vi "Do.vi"(8 "error in (no error)":errorcluster, 10 "Actor in":refnum<class "Actor.lvclass">, 11 "Configure Output Mode Msg":refnum<class "Configure Output Mode Msg.lvclass">) -> (0 "error out":errorcluster, 2 "Actor out":refnum<class "Actor.lvclass">)   [LabVIEW 2015, in "CS++Fgen.lvlib" / "Configure Output Mode Msg.lvclass"]
doc: "This VI delivers the message to the actor by calling the appropriate method(s) on the actor."
uses:
  Configure Output Mode Msg.lvclass
  <vilib>/ActorFramework/Actor/Actor.lvclass
  CS++Fgen/CS++Fgen.lvclass
  CSPP_Core/Actors/CS++PVMonitor Messages/CS++PVUpdate Msg/CS++PVUpdate Msg.lvclass/CS++PVUpdate Msg.ctl
  CSPP_Core/Classes/CS++ProcessVariables/ProcessVariable/PV.lvclass/PV.ctl
  Configure Output Mode Msg.lvclass/Configure Output Mode Msg.ctl
  CSPP_Core/Classes/CS++ProcessVariables/ProcessVariable/PV.lvclass
  CSPP_Core/Actors/CS++PVMonitor Messages/CS++PVUpdate Msg/CS++PVUpdate Msg.lvclass
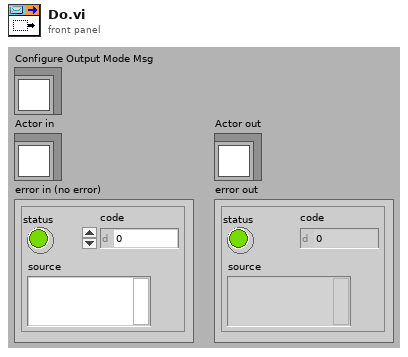
[diagram p1: front panel]
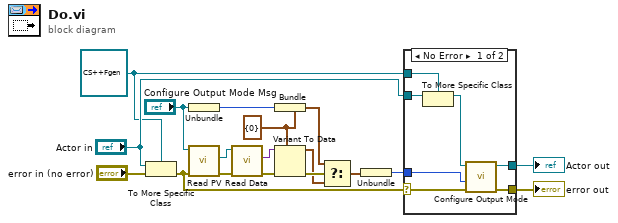
[diagram p0: block diagram]
diagram:
  w10 = cluster{"output mode (Standard Function)":i32} {"output mode (Standard Function)"=0} ("Type")
  w14 = refnum<class "CS++Fgen.lvclass"> refnum ("Actor in")
  n1 = To More Specific Class(target class=w14, reference="Actor in", error in="error in (no error)") -> (error out=w3:errorcluster)  [unwired: 1 out]
  n2 = Unbundle ("Pre-Unbundler")("Configure Output Mode Msg") -> (w1:i32)
  n3 = call "Read PV.vi"("error in (no error)"=w3, "CS++PVUpdate Msg in"="Configure Output Mode Msg") -> ("error out"=w13:errorcluster, "PV"=w9:refnum<class "PV.lvclass">)  [unwired: 7 in, 1 out]
  n4 = call "Read Data.vi"("error in (no error)"=w13, "PV in"=w9) -> ("error out"=w7:errorcluster, "Data"=w8:variant)  [unwired: 7 in, 1 out]
  n5 = Bundle ("Pre-Bundler")(cluster=w10, "output mode (Standard Function)"=w1) -> (w11:cluster{"output mode (Standard Function)":i32})
  n6 = Variant To Data(error in=w7, type=w10, Variant=w8) -> (data=w5:cluster{"output mode (Standard Function)":i32}, error out=w12:errorcluster)
  n7 = Select ("MainSelect")(t=w11, s=w12, f=w5) -> (s? t:f=w6:cluster{"output mode (Standard Function)":i32})
  n8 = Unbundle ("Main-Unbundler")(w6) -> ("output mode (Standard Function)"=w2:i32)
  n9 = case shown="No Error" w3 {
    selector: w3 -> [w23 w27]
    tunnel: [w25 w27] -> w17
    tunnel: [w24 w26] -> w16
    tunnel: "Actor in" -> [w22 w26]
    tunnel: w14 -> [w21 _]
    tunnel: w2 -> [w19 _]
    frame No Error {
      n10 = To More Specific Class(target class=w21, reference=w22) -> (specific class reference=w20:refnum<class "CS++Fgen.lvclass">)  [unwired: 1 in, 1 out]
      n11 = call "Configure Output Mode.vi"("error in (no error)"=w23, "output mode (Standard Function)"=w19, "CS++Fgen in"=w20) -> ("error out"=w25:errorcluster, "CS++Fgen out"=w24:refnum<class "CS++Fgen.lvclass">)  [unwired: 7 in]
    }
    frame Error {
    }
  }
  "error out" <- w17
  "Actor out" <- w16
